vi "Delete Default Value.vi"(4 "label or caption":string) -> (1 "naked label or caption":string)   [LabVIEW 2018, in "NISAST VI Scripting.lvlib" / "VI.lvlib" / "Front Panel.lvlib"]
uses:
  Front Panel.lvlib
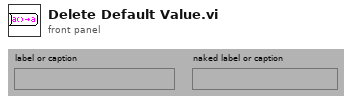
[diagram p1: front panel]
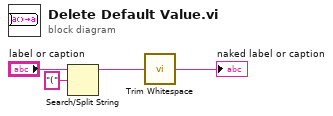
[diagram p0: block diagram]
diagram:
  n1 = Search/Split String(string="label or caption", search string/char (-)="(") -> (substring before match=w2:string)  [unwired: 3 out]
  n2 = call <vilib>:"Trim Whitespace.vi"("string"=w2) -> ("trimmed string"=→"naked label or caption":string)  [unwired: 1 in]
